vi "ATF-Error FGV.vi"(7 "Enum":enum16{"Read", "Write", "Clear"}(ring), 11 "CS err":T1) -> (3 "CS err":T1)   [LabVIEW 2022 SP3]
uses:
  327e6077-3b0d-4314-8121-d1810440615f.vi
panel:
  out "s? t:f":string
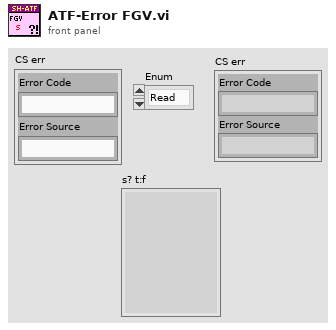
[diagram p1: front panel]
types:
  T1 = cluster{"Error Code":string, "Error Source":string}
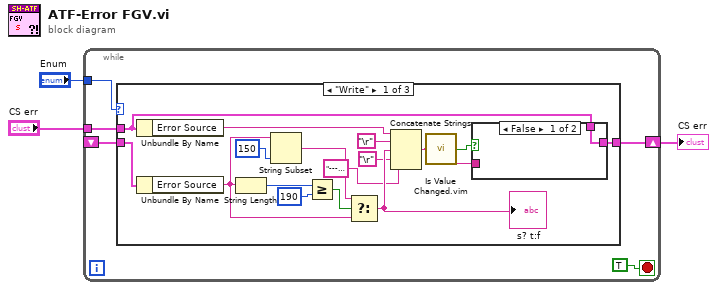
[diagram p0: block diagram]
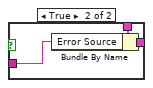
[diagram p2: hidden frame]
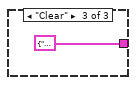
[diagram p4: hidden frame]
diagram:
  n1 = while {
    tunnel: "Enum" -> [w8]
    tunnel: "CS err" -> [w7]
    shift-right: [w6] -> w3
    shift-left: _ -> [w5]
    stop <- TRUE stop-if-true
    n2 = case shown="\"Write\"" w8 {
      tunnel: w7 -> [w22 _ _]
      tunnel: [w23 w29 T1 {"Error Code"="", "Error Source"=""} ("RT Error")] -> w6
      tunnel: w5 -> [w15 w29 _]
      frame "Write" {
        n3 = Unbundle By Name(w22) -> ("Error Source"=w24:string)
        n4 = Unbundle By Name(w15) -> ("Error Source"=w13:string)
        n5 = String Length(string=w13) -> (length=w19:i32)
        n6 = String Subset(string=w13, length (rest)=150 ("length (rest)")) -> (substring=w16:string)  [unwired: 1 in]
        n7 = Greater Or Equal?(x=w19, y=190) -> (x >= y?=w20:bool)
        n8 = Select(t=w16, s=w20, f=w13) -> (s? t:f=w14:string)
        "s? t:f" <- w14
        n9 = Concatenate Strings(w24, "\r", w14, "\r", "------------" ("string")) -> (w9:string)
        n10 = call "Is Value Changed.vim"("value"=w9) -> ("changed or first call?"=w10:bool)
        n11 = case shown="False" w10 {
          tunnel: [w25 w28] -> w23
          tunnel: w22 -> [w25 w27]
          tunnel: w9 -> [_ w26]
          frame False {
          }
          frame True {
            n12 = Bundle By Name(cluster=w27, "Error Source"=w26) -> (w28:T1)
          }
        }
      }
      frame "Read", Default {
      }
      frame "Clear" {
      }
    }
  }
  "CS err" <- w3
